vi "Write MethodRefnum.vi"(8 "error in (no error)":errorcluster, 10 "MethodRefnum":refnum<vi>, 11 "CS++Methods in":refnum<class "CS++Method.lvclass">) -> (0 "error out":errorcluster, 3 "CS++Methods out":refnum<class "CS++Method.lvclass">)   [LabVIEW 2016, in "CS++Method.lvlib" / "CS++Method.lvclass"]
uses:
  CS++Method.lvclass
  CS++Method.lvclass/CS++Method.ctl
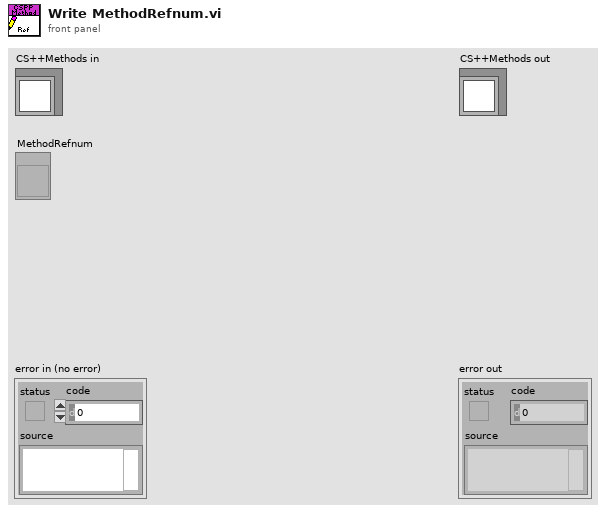
[diagram p1: front panel]
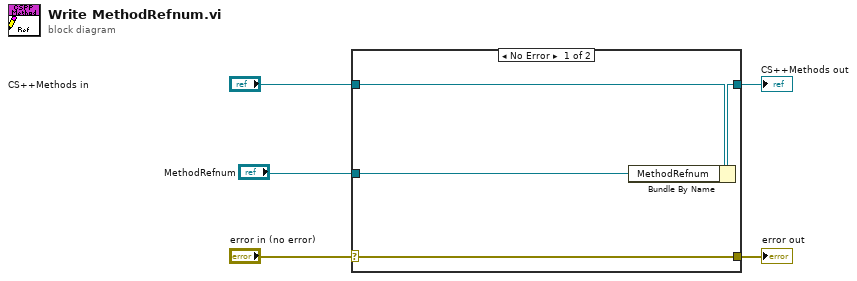
[diagram p0: block diagram]
diagram:
  n1 = case shown="No Error" "error in (no error)" {
    selector: "error in (no error)" -> [w9 w10]
    tunnel: [w9 w10] -> w4
    tunnel: [w7 w11] -> w2
    tunnel: "CS++Methods in" -> [w8 w11]
    tunnel: "MethodRefnum" -> [w6 _]
    frame No Error {
      n2 = Bundle By Name(cluster=w8, "MethodRefnum"=w6) -> (w7:refnum<class "CS++Method.lvclass">)
    }
    frame Error {
    }
  }
  "error out" <- w4
  "CS++Methods out" <- w2
